vi "Start.vi"(8 "error in (no error)":errorcluster, 11 "Motor in":refnum<class "Motor.lvclass">) -> (0 "error out":errorcluster, 3 "Motor out":refnum<class "Motor.lvclass">)   [LabVIEW 2013, in "PowderDeposition.lvlib" / "Motor.lvclass"]
uses:
  Motor.lvclass
  Main/Custom-errors.ctl
  Main/PD-Main.lvclass
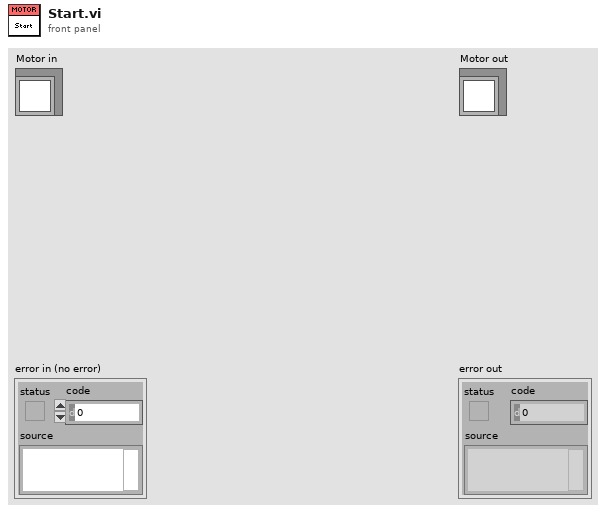
[diagram p1: front panel]
types:
  T1 = typedef "PowderDeposition.lvlib/PD-Main.lvclass/Custom-errors.ctl" = enum16{"Not implemented", "Command not recognized", "Invalid input", "Timeout", "Load file failed", "Action failed", "Action invalid", "Motor inactive", "Not in range", "Unsafe state"}
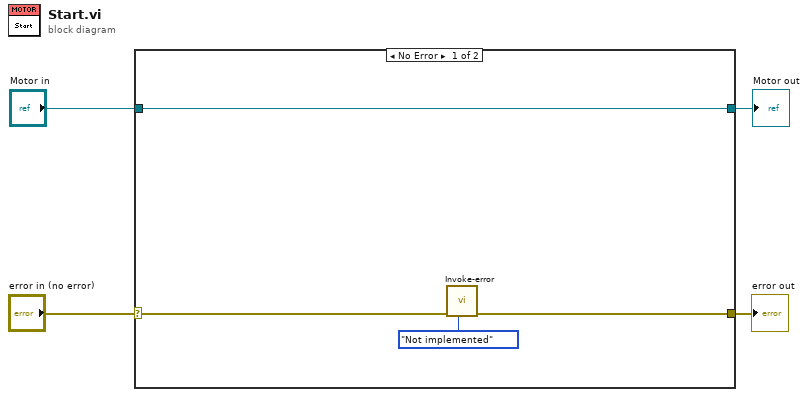
[diagram p0: block diagram]
diagram:
  n1 = case shown="No Error" "error in (no error)" {
    selector: "error in (no error)" -> [w6 w10]
    tunnel: [w5 w10] -> w3
    tunnel: [w8 w9] -> w1
    tunnel: "Motor in" -> [w8 w9]
    frame No Error {
      n2 = call "Invoke-error.vi"("Error"=Custom-errors."Not implemented", "error in (no error)"=w6) -> ("error out"=w5:errorcluster)  [unwired: 9 in]
    }
    frame Error {
    }
  }
  "error out" <- w3
  "Motor out" <- w1
